vi "resample.vi"(8 "error in (no error)":errorcluster, 9 "Height":i32, 10 "Width":i32, 11 "Image in":T1) -> (0 "error out":errorcluster, 3 "Image out":T1)   [LabVIEW 2022 SP3, in "Vision.lvlib"]
uses:
  Vision.lvlib
  <vilib>/vision/Image Controls.llb/IMAQ Image.ctl
  bin/Vision.dll
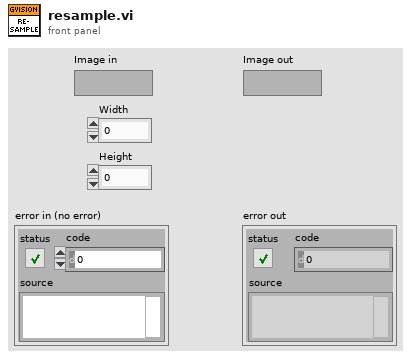
[diagram p1: front panel]
types:
  T1 = typedef "IMAQ Image.ctl" = refnum<image>
  T2 = enum32{"Map Pixel Pointer", "Unmap Pixel Pointer", "Get Pixels Infos"}
  T3 = typedef "Image Type" = u32
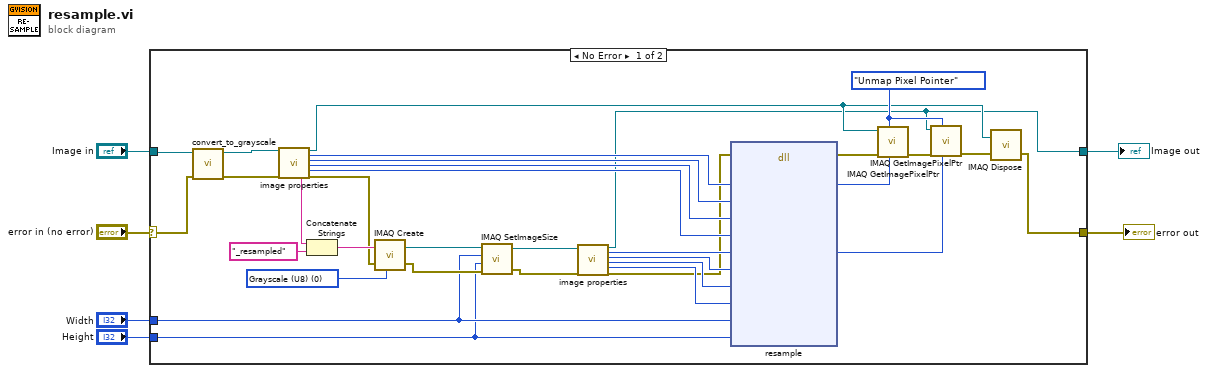
[diagram p0: block diagram]
diagram:
  n1 = case shown="No Error" "error in (no error)" {
    selector: "error in (no error)" -> [w29 w41]
    tunnel: "Image in" -> [w31 w40]
    tunnel: [w39 w41] -> w4
    tunnel: [w7 w40] -> w3
    tunnel: "Width" -> [w15 _]
    tunnel: "Height" -> [w14 _]
    frame No Error {
      w32 = T2."Unmap Pixel Pointer" ("Function")
      w36 = T3 0 items=["Grayscale (U8)", "Grayscale (I16)", "Grayscale (SGL)", "Complex (CSG)", "RGB (U32)", "HSL (U32)", "RGB (U64)", "Grayscale (U16)"] ("Image Type")
      n2 = call "convert_to_grayscale.vi"("error in (no error)"=w29, "Image in"=w31) -> ("error out"=w28:errorcluster, "Image out"=w30:T1)  [unwired: 8 in]
      n3 = call "image properties.vi"("Image in"=w30, "error in (no error)"=w28) -> ("Image Name"=w27:string, "Image out"=w10:T1, "Pixel Pointer out"=w26:u64, "Line Width"=w25:i32, "X Resolution"=w24:i32, "Y Resolution"=w23:i32, "error out"=w18:errorcluster)  [unwired: 11 in]
      n4 = Concatenate Strings(w27, "_resampled" ("string")) -> (w37:string)
      n5 = call "IMAQ Create"("Image Name"=w37, "Image Type"=w36, "error in (no error)"=w18) -> ("New Image"=w17:T1, "error out"=w16:errorcluster)  [unwired: 2 in]
      n6 = call "IMAQ SetImageSize"("error in (no error)"=w16, "Y Resolution"=w14, "X Resolution"=w15, "Image"=w17) -> ("error out"=w12:errorcluster, "Image Out"=w13:T1)  [unwired: 1 in]
      n7 = call "image properties.vi"("Image in"=w13, "error in (no error)"=w12) -> ("Image out"=w7:T1, "Pixel Pointer out"=w22:u64, "Line Width"=w21:i32, "X Resolution"=w20:i32, "Y Resolution"=w19:i32, "error out"=w11:errorcluster)  [unwired: 11 in, 1 out]
      n8 = dll-call lib="C:/Users/Caleb/Desktop/nebraska-silicon-lab/pixel-gantry-control/Gantry/Shared Components/External/bin/Vision.dll" fn="resample"(error in=w11, "src_imgPtr"=w26, "src_imgLineWidth"=w25, "src_imgWidth"=w24, "src_imgHeight"=w23, "dst_imgPtr"=w22, "dst_imgLineWidth"=w21, "dst_imgWidth"=w20, "dst_imgHeight"=w19, "new_width"=w15, "new_height"=w14) -> (error out=w34:errorcluster, "src_imgPtr"=w9:u64, "dst_imgPtr"=w8:u64)  [unwired: 11 in, 1 out]
      n9 = call "IMAQ GetImagePixelPtr"("Pixel Pointer in"=w9, "Function"=w32, "error in (no error)"=w34, "Image"=w10) -> ("error out"=w35:errorcluster)  [unwired: 2 in, 5 out]
      n10 = call "IMAQ GetImagePixelPtr"("Pixel Pointer in"=w8, "Function"=w32, "error in (no error)"=w35, "Image"=w7) -> ("error out"=w33:errorcluster)  [unwired: 2 in, 5 out]
      n11 = call "IMAQ Dispose"("Image"=w10, "error in (no error)"=w33) -> ("error out"=w39:errorcluster)  [unwired: 4 in]
    }
    frame Error {
    }
  }
  "Image out" <- w3
  "error out" <- w4
